vi "On Save File Security Check Starting.vi"(8 "error in (no error)":errorcluster, 10 "Data":T1, 11 "WebView2 Event Filter Interface in":refnum<class "WebView2 Event Filter Interface.lvclass">) -> (0 "error out":errorcluster, 1 "SuppressDefaultPolicy":bool, 2 "CancelSave":bool)   [LabVIEW 2025, in "WebView2.lvlib" / "WebView2 Event Filter Interface.lvclass"]
uses:
  WebView2 Event Filter Interface.lvclass
  WebView2 Control Object/Save File Security Check Starting Event Data.ctl
  WebView2 Control Object/WebView2 Control.lvclass
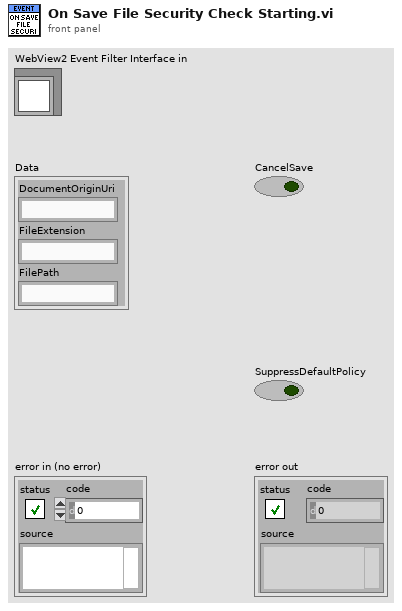
[diagram p1: front panel]
types:
  T1 = typedef "WebView2.lvlib/WebView2 Control.lvclass/Save File Security Check Starting Event Data.ctl" = cluster{"DocumentOriginUri":string, "FileExtension":string, "FilePath":string}
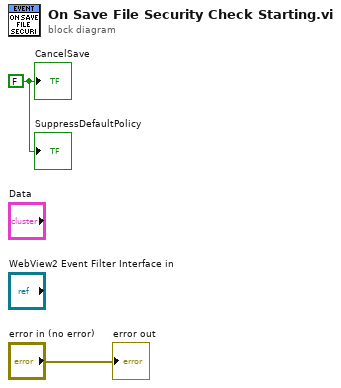
[diagram p0: block diagram]
diagram:
  w1 = FALSE ("CancelSave")
  "error out" <- "error in (no error)"
  "CancelSave" <- w1
  "SuppressDefaultPolicy" <- w1
